vi "BuildCall.vi"(7 "PythonConverter_BD in":refnum<class "PyConvBD.lvclass">, 8 "error in":errorcluster, 11 "Node in":refnum<class "Node.lvclass">) -> (0 "error out":errorcluster, 3 "Node out":refnum<class "Node.lvclass">, 5 "PythonConverter_BD out":refnum<class "PyConvBD.lvclass">)   [LabVIEW 2014, in "Node.lvclass"]
uses:
  Node.lvclass
  Python/PythonConverter_BD/PyConvBD.lvclass
  Python/PythonConverter_BD/TypeDefs/NodeCall_TD.ctl
  Python/Parsing/ListTypesTD.ctl
  Python/Parsing/Classes/PythonFunction/PythonFunction.lvclass/PythonFunction.ctl
  Python/Parsing/Classes/PythonFunction/PythonFunction.lvclass
  Python/Parsing/Python Functions.lvlib
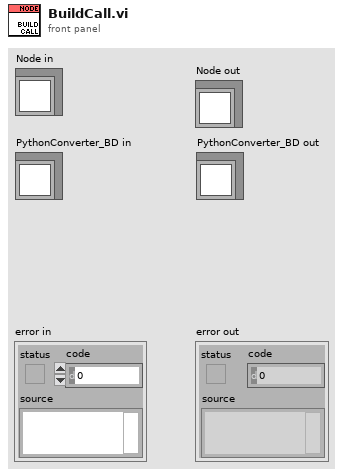
[diagram p1: front panel]
types:
  T1 = typedef "Python Functions.lvlib/ListTypesTD.ctl" = enum16{"list", "tuple", "parameter list", "output list"}
  T2 = typedef "NodeCall_TD.ctl" = cluster{"call":string, "collect":string, "Threaded":bool, "branches":string[]}
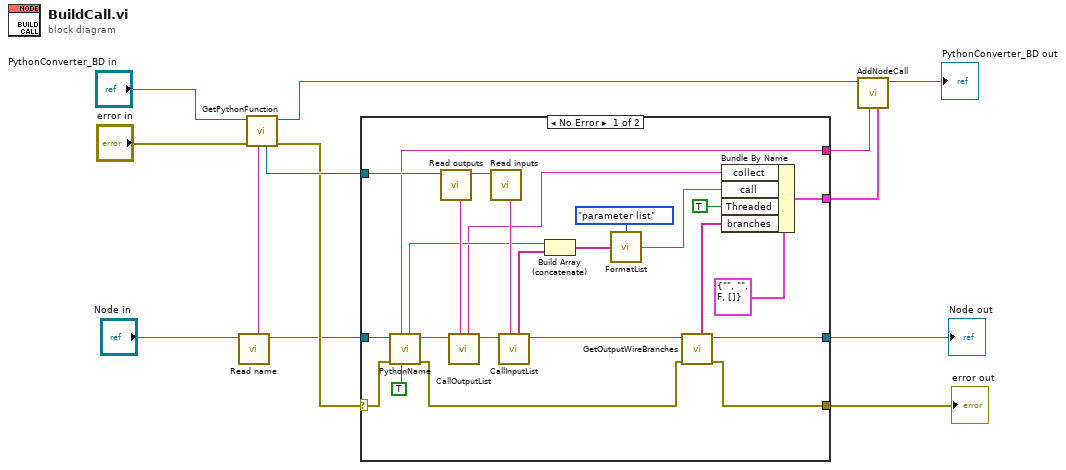
[diagram p0: block diagram]
diagram:
  n1 = call-dynamic "Read name.vi"("Node in"="Node in") -> ("Node out"=w7:refnum<class "Node.lvclass">, "name"=w8:string)  [unwired: 7 in]
  n2 = call "GetPythonFunction.vi"("function name"=w8, "error in"="error in", "PythonConverter_BD in"="PythonConverter_BD in") -> ("error out"=w12:errorcluster, "PythonConverter_BD out"=w11:refnum<class "PyConvBD.lvclass">, "Python function"=w13:refnum<class "PythonFunction.lvclass">)  [unwired: 4 in]
  n3 = case shown="No Error" w12 {
    selector: w12 -> [w33 w39]
    tunnel: [w17 w39] -> w4
    tunnel: [w25 _] -> w10
    tunnel: w7 -> [w32 w38]
    tunnel: w13 -> [w35 _]
    tunnel: [w31 _] -> w9
    tunnel: [w19 w38] -> w5
    frame No Error {
      n4 = call-dynamic "PythonName.vi"("add self"=TRUE, "error in"=w33, "Node in"=w32) -> ("error out"=w18:errorcluster, "Node out"=w15:refnum<class "Node.lvclass">, "name"=w30:string, "UID"=w31:string)  [unwired: 5 in]
      n5 = call "Read outputs.vi"("PythonFunction in"=w35) -> ("PythonFunction out"=w34:refnum<class "PythonFunction.lvclass">, "outputs"=w37:string)  [unwired: 7 in]
      n6 = call-dynamic "CallOutputList.vi"("list"=w37, "Node in"=w15) -> ("Node out"=w14:refnum<class "Node.lvclass">, "call outputs"=w22:string)  [unwired: 6 in]
      n7 = call "Read inputs.vi"("PythonFunction in"=w34) -> ("inputs"=w36:string)  [unwired: 7 in, 1 out]
      n8 = call-dynamic "CallInputList.vi"("list"=w36, "Node in"=w14) -> ("Node out"=w20:refnum<class "Node.lvclass">, "call inputs"=w29:string[])  [unwired: 6 in]
      n9 = Build Array (concatenate)(w30, w29) -> (w23:string[])
      n10 = call "FormatList.vi"("values"=w23, "type"=ListTypesTD."parameter list") -> ("python object"=w21:string)
      n11 = call-dynamic "GetOutputWireBranches.vi"("error in"=w18, "Node in"=w20) -> ("error out"=w17:errorcluster, "Node out"=w19:refnum<class "Node.lvclass">, "branches"=w16:string[])  [unwired: 5 in]
      n12 = Bundle By Name(cluster=T2 {"call"="", "collect"="", "Threaded"=FALSE, "branches"=[]} ("call"), "collect"=w22, "call"=w21, "Threaded"=TRUE, "branches"=w16) -> (w25:T2)
    }
    frame Error {
    }
  }
  "error out" <- w4
  "Node out" <- w5
  n13 = call "AddNodeCall.vi"("call"=w10, "name"=w9, "PythonConverter_BD in"=w11) -> ("PythonConverter_BD out"=→"PythonConverter_BD out":refnum<class "PyConvBD.lvclass">)  [unwired: 5 in, 1 out]
